vi "DVR.same.Write.vi"(8 "error in":errorcluster, 10 "save.same?":bool, 11 "DVR in":T1) -> (0 "error out":errorcluster)   [LabVIEW 2020]
uses:
  _controls/data.ctl
  camera/camera.lvclass
  _controls/data.ref.ctl
  <vilib>/vision/Image Controls.llb/IMAQ Image.ctl
  _controls/state.ctl
  _controls/data.vars.ctl
  _controls/flip.ctl
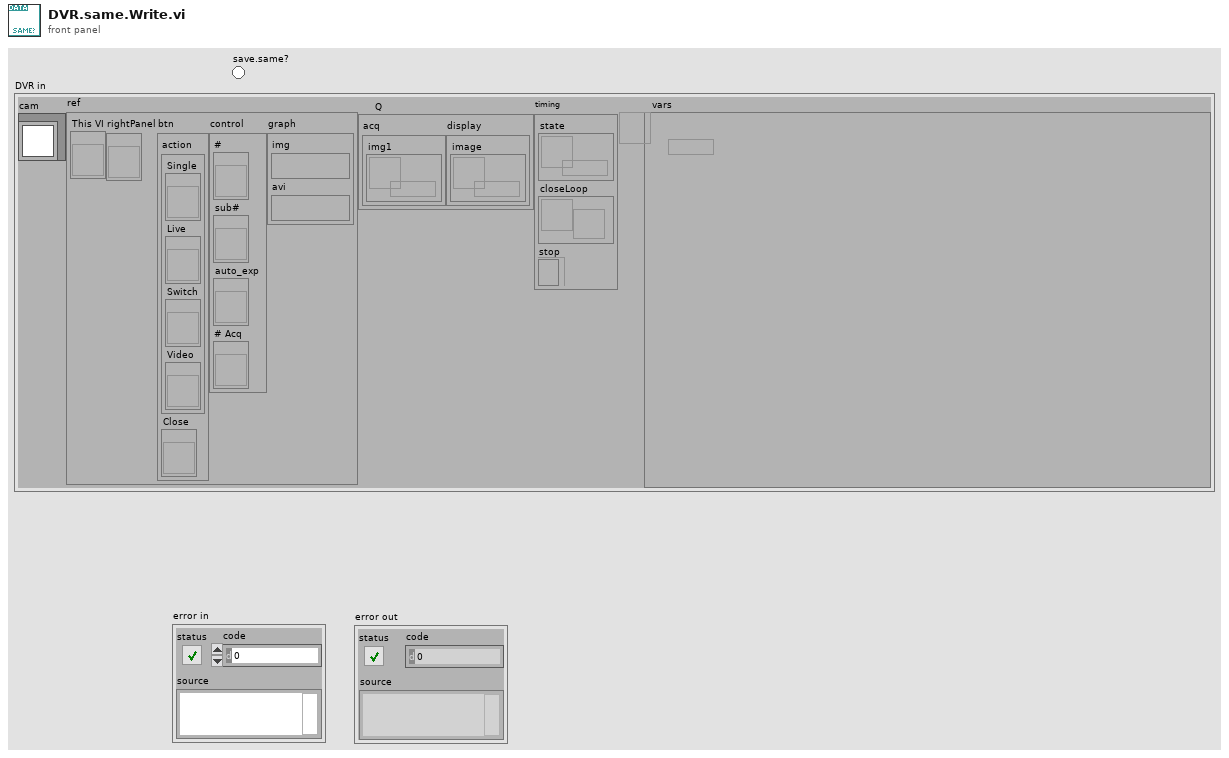
[diagram p1: front panel]
types:
  T1 = typedef "data.ctl" = cluster{"cam":refnum<class "camera.lvclass">, "ref":T2, "Q":cluster{"acq":cluster{"img1":refnum<queue>}, "display":cluster{"image":refnum<queue>}}, "timing":cluster{"state":refnum<queue>, "closeLoop":refnum<notifier>, "stop":refnum<k4>}, "vars":refnum<data-value>}
  T2 = typedef "data.ref.ctl" = cluster{"This VI":refnum<vi>, "rightPanel":refnum<vi>, "btn":cluster{"action":cluster{"Single":refnum<vi>, "Live":refnum<vi>, "Switch":refnum<vi>, "Video":refnum<vi>}, "Close":refnum<vi>}, "control":cluster{"#":refnum<vi>, "sub#":refnum<vi>, "auto_exp":refnum<vi>, "# Acq":refnum<vi>}, "graph":cluster{"img":T3, "avi":T3}}
  T3 = typedef "IMAQ Image.ctl" = refnum<image>
  T4 = typedef "data.vars.ctl" = cluster{"save":cluster{"base_folder":cluster{"Folder":path, "tif":bool, "jpg":bool}, "module":string, "#":u32, "sub#":u8, "save.op":enum16{"Full", "Light"}, "same?":bool, "Shift":enum16{"Single", "Leapfrog"}, "jpg?":bool, "flip":T5}, "acq":cluster{"# Acq":u16, "rotate":bool, "FPS":dbl}, "calib.manual":cluster{"BG":cluster{"Image":u16[][], "enabled?":bool}, "FF":cluster{"Image":u16[][], "enabled?":bool}}}
  T5 = typedef "flip.ctl" = cluster{"x":bool, "y":bool}
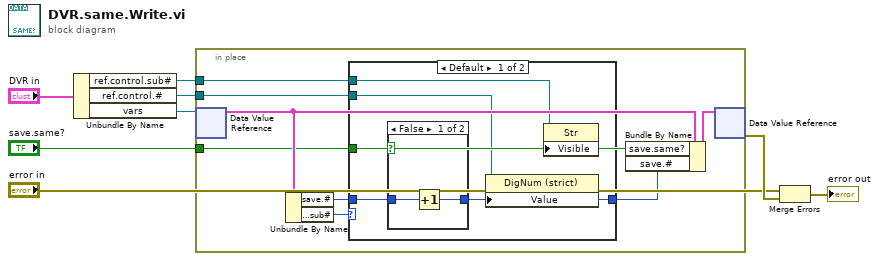
[diagram p0: block diagram]
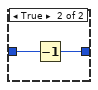
[diagram p2: hidden frame]
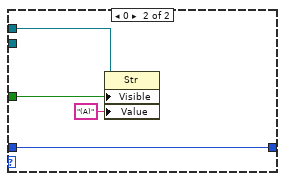
[diagram p3: hidden frame]
diagram:
  n1 = Unbundle By Name("DVR in") -> ("ref.control.sub#"=w2:refnum<vi>, "ref.control.#"=w1:refnum<vi>, "vars"=w7:refnum<data-value>)
  n2 = in-place {
    in-place-border: "save.same?" -> [w10]
    in-place-border: w2 -> [w13]
    in-place-border: w1 -> [w9]
    n3 = in-place-dvr #1(w7) -> (w14:T4)  [unwired: 1 out]
    n4 = Unbundle By Name(w14) -> ("save.#"=w12:u32, "save.sub#"=w15:u8)
    n5 = case shown="Default" w15 {
      tunnel: w13 -> [w18 w26]
      tunnel: w12 -> [w21 w29]
      tunnel: [w19 w29] -> w11
      tunnel: w10 -> [w17 w28]
      tunnel: w9 -> [w20 _]
      frame Default {
        n6 = case shown="False" w17 {
          tunnel: w21 -> [w23 w25]
          tunnel: [w22 w24] -> w19
          frame False {
            n7 = Increment(x=w23) -> (x+1=w22:u32)
          }
          frame True {
            n8 = Decrement(x=w25) -> (x-1=w24:u32)
          }
        }
        n9 = property class="DigNum (strict)"(reference=w20, "Value"=w19) -> ()  [unwired: 1 in, 2 out]
        n10 = property class="Str"(reference=w18, "Visible"=w17) -> ()  [unwired: 1 in, 2 out]
      }
      frame 0 {
        n11 = property class="Str"(reference=w26, "Visible"=w28, "Value"="(A)") -> ()  [unwired: 1 in, 2 out]
      }
    }
    n12 = Bundle By Name(cluster=w14, "save.same?"=w10, "save.#"=w11) -> (w16:T4)
    n13 = in-place-dvr #1(w16) -> (w8:errorcluster)  [unwired: 1 out]
  }
  n14 = Merge Errors("error in", w8) -> (→"error out":errorcluster)
